vi "_RT_CtrlLoop_DigitalAnalogueOutput.vi"(6 "ExpVar.lvclass":refnum<class "ExpVar.lvclass">, 8 "error in (no error)":errorcluster, 9 "safty":refnum<data-value>) -> ()   [LabVIEW 2018]
uses:
  PublicSubVI/NewExpVar/ExpVar.lvclass
  PublicSubVI/Ctl/_ctl_RT_FPGA_Function.ctl
  PublicSubVI/Ctl/_ctl_RT_extDO.ctl
  PublicSubVI/Ctl/_ctl_RT_ExtAO.ctl
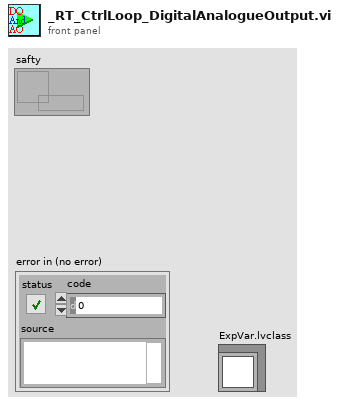
[diagram p1: front panel]
types:
  T1 = enum16{"None", "D999", "ExtAO", "ExtDO", "ExtDI_Label", "Signal_Remarks", "Script"}
  T2 = typedef "_ctl_RT_FPGA_Function.ctl" = enum16{"Initialisation", "Execution", "Digital In"}
  T3 = enum16{"via string label", "Laser", "Pressure", "TMP", "Script", "Signal Remarks", "ExtAO", "ExtDO", "ExtDI", "D999"}
  T4 = typedef "_ctl_RT_extDO.ctl" = cluster{"Label":string, "Boolean":bool}[]
  T5 = typedef "_ctl_RT_ExtAO.ctl" = cluster{"Label":string, "y":dbl}[]
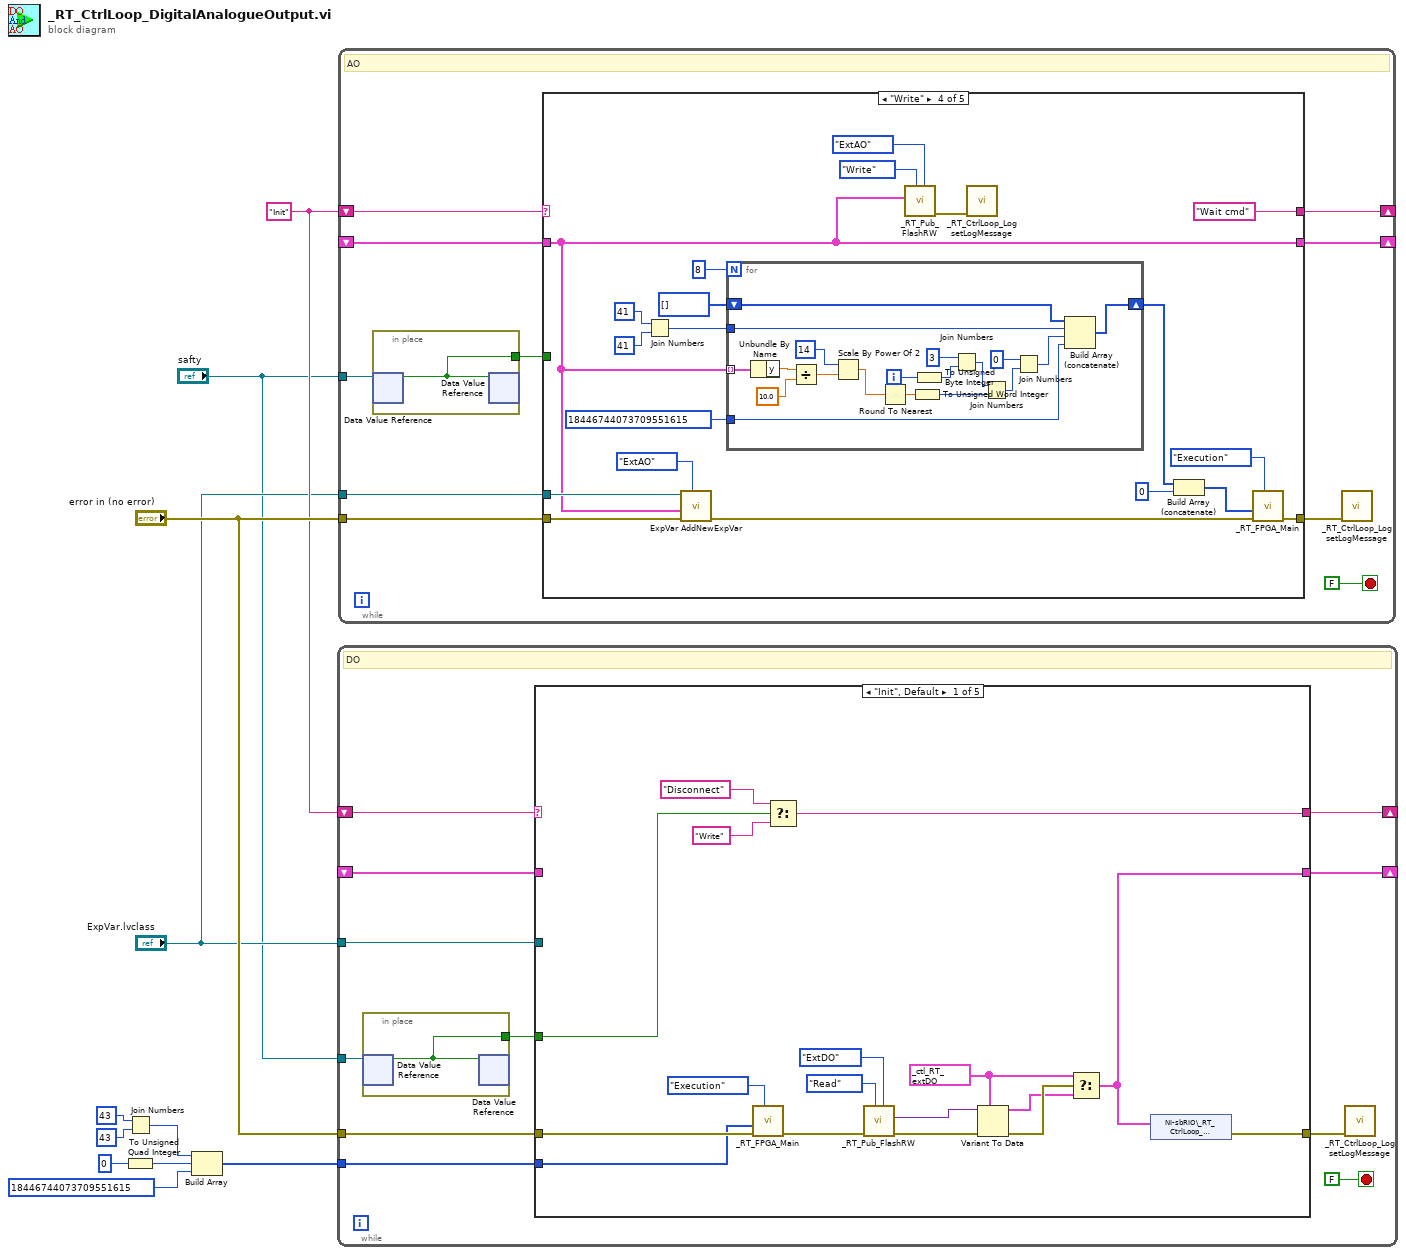
[diagram p0: block diagram]
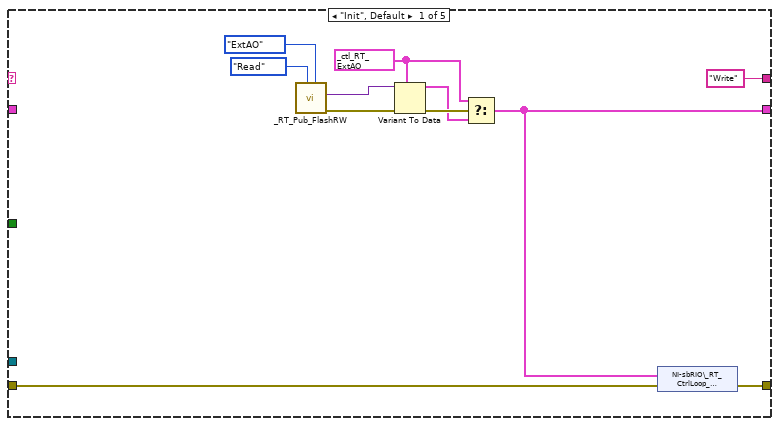
[diagram p2: hidden frame]
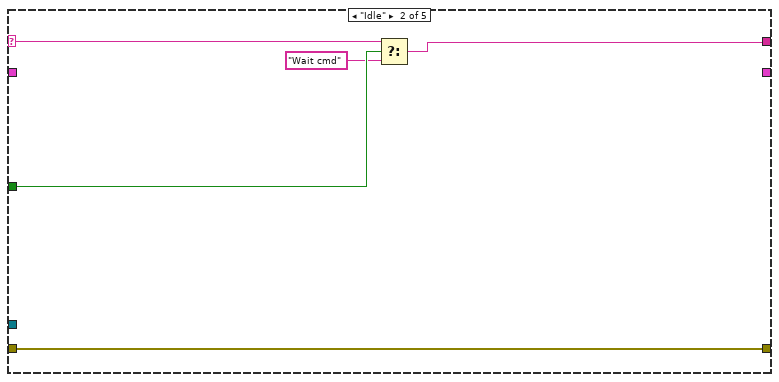
[diagram p3: hidden frame]
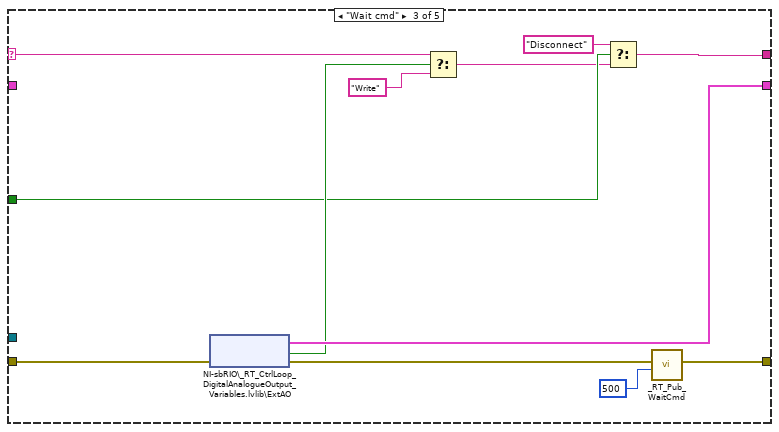
[diagram p4: hidden frame]
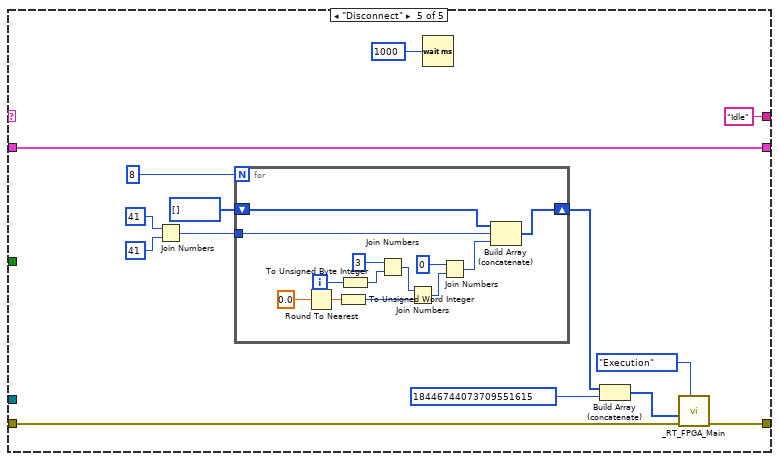
[diagram p5: hidden frame]
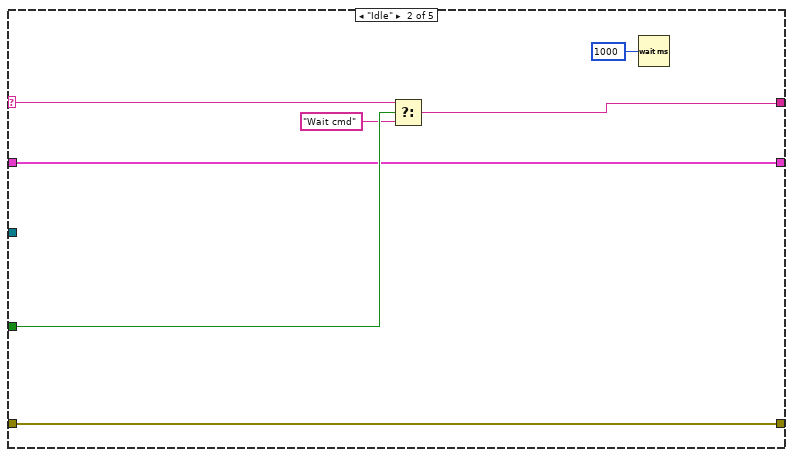
[diagram p6: hidden frame]
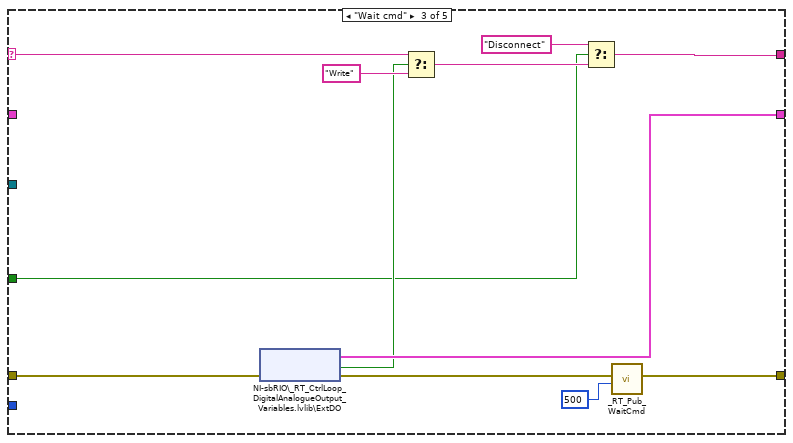
[diagram p7: hidden frame]
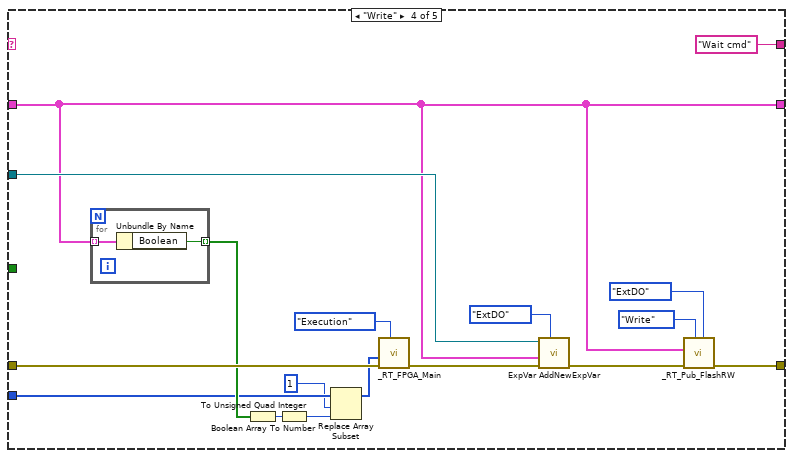
[diagram p8: hidden frame]
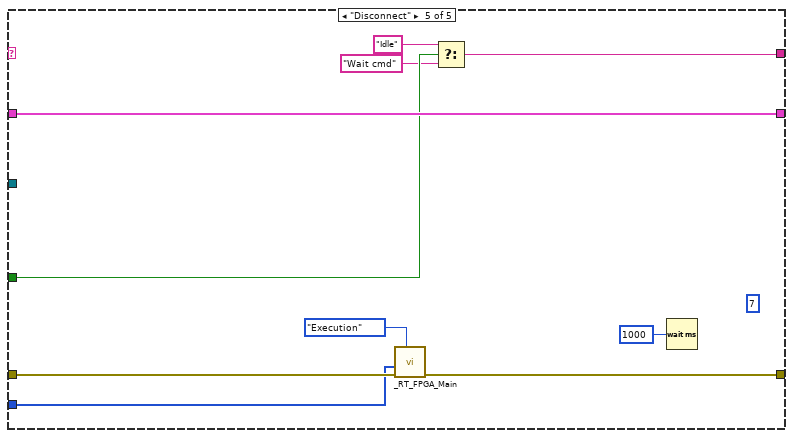
[diagram p9: hidden frame]
diagram:
  w3 = "Init"
  n1 = To Unsigned Quad Integer(1:u64 0 ("number")) -> (0:w7:u64)
  n2 = Join Numbers(hi=u32 43, lo=u32 43) -> ((hi.lo)=w10:u64)
  n3 = Build Array(w10, w7, u64 18446744073709551615 ("element")) -> (w4:u64[])
  n4 = while {
    shift-right: [w17] -> _
    shift-left: w3 -> [w19]
    shift-right: [w22] -> _
    shift-left: _ -> [w21]
    tunnel: "error in (no error)" -> [w20]
    tunnel: w4 -> [w16]
    tunnel: "ExpVar.lvclass" -> [w15]
    tunnel: "safty" -> [w13]
    stop <- FALSE stop-if-true
    # "DO"
    n5 = in-place {
      in-place-border: [w23] -> w12
      n6 = in-place-dvr #1(w13) -> (w23:bool)  [unwired: 1 out]
      n7 = in-place-dvr #1(w23) -> ()  [unwired: 2 out]
    }
    n8 = case shown="\"Init\", Default" w19 {
      selector: w19 -> [_ w41 w51 _ _]
      tunnel: [w36 w46 w48 "Wait cmd" w83] -> w17
      tunnel: [w25 w45 w55 w63 w86] -> w22
      tunnel: w21 -> [_ w45 _ w63 w86]
      tunnel: w20 -> [w35 w44 w59 w74 w87]
      tunnel: [w39 w44 w58 w61 w84] -> w14
      tunnel: w16 -> [w34 _ _ w71 w85]
      tunnel: w15 -> [_ _ _ w67 _]
      tunnel: w12 -> [w24 w47 w49 _ w80]
      frame "Init", Default {
        w26 = T4 [{"Label"="DO0", "Boolean"=FALSE}, {"Label"="DO1", "Boolean"=FALSE}, {"Label"="DO2", "Boolean"=FALSE}, {"Label"="DO3", "Boolean"=FALSE}, {"Label"="DO4", "Boolean"=FALSE}, {"Label"="DO5", "Boolean"=FALSE}, {"Label"="DO6", "Boolean"=FALSE}, {"Label"="DO7", "Boolean"=FALSE}] ("DOs")
        n9 = call "_RT_FPGA_Main.vi"("Function"=_ctl_RT_FPGA_Function."Execution", "Error in"=w35, "U64EventCodes"=w34) -> ("Error out"=w32:errorcluster)  [unwired: 6 in, 2 out]
        n10 = Select(t="Disconnect", s=w24, f="Write") -> (s? t:f=w36:string)
        n11 = call "_RT_Pub_FlashRW.vi"("FileEnum"=T1."ExtDO", "State"=enum16{"Read", "Write"}."Read", "error in (no error)"=w32) -> ("error out"=w30:errorcluster, "Value"=w31:variant)  [unwired: 6 in, 1 out]
        n12 = Variant To Data(error in=w30, type=w26, Variant=w31) -> (data=w27:T4, error out=w28:errorcluster)
        n13 = Select(t=w26, s=w28, f=w27) -> (s? t:f=w25:T4)
        n14 = shared-variable "NI-sbRIO\\_RT_CtrlLoop_DigitalAnalogueOutput_Variables.lvlib\\ExtDO"(w25) -> (error out=w39:errorcluster)  [unwired: 1 in]
      }
      frame "Idle" {
        n15 = Select(t=w41, s=w47, f="Wait cmd") -> (s? t:f=w46:string)
        n16 = Wait (ms)(milliseconds to wait=u32 1000) -> ()  [unwired: 1 out]
      }
      frame "Wait cmd" {
        n17 = shared-variable "NI-sbRIO\\_RT_CtrlLoop_DigitalAnalogueOutput_Variables.lvlib\\ExtDO"(error in=w59) -> (w55:T4, error out=w57:errorcluster, w50:bool)  [unwired: 1 in]
        n18 = Select(t=w51, s=w50, f="Write") -> (s? t:f=w52:string)
        n19 = Select(t="Disconnect", s=w49, f=w52) -> (s? t:f=w48:string)
        n20 = call "_RT_Pub_WaitCmd.vi"("milliseconds to wait"=u32 500, "error in (no error)"=w57) -> ("error out"=w58:errorcluster)  [unwired: 9 in]
      }
      frame "Write" {
        n21 = for {
          tunnel: w63 -> [w78] mode=indexing
          tunnel: [w77] -> w72 mode=indexing
          n22 = Unbundle By Name(w78) -> ("Boolean"=w77:bool)
        }
        n23 = Boolean Array To Number(Boolean array=w72) -> (number=w73:u32)
        n24 = To Unsigned Quad Integer(1:w73) -> (0:w69:u64)
        n25 = Replace Array Subset(array=w71, new element=w69, index=1) -> (w68:u64[])
        n26 = call "_RT_FPGA_Main.vi"("Function"=_ctl_RT_FPGA_Function."Execution", "Error in"=w74, "U64EventCodes"=w68) -> ("Error out"=w66:errorcluster)  [unwired: 6 in, 2 out]
        n27 = call-dynamic "ExpVar AddNewExpVar.vi"("VarType"=T3."ExtDO", "error in (no error)"=w66, "Var"=w63, "ExpVar in"=w67) -> ("error out"=w62:errorcluster)  [unwired: 6 in, 1 out]
        n28 = call "_RT_Pub_FlashRW.vi"("FileEnum"=T1."ExtDO", "State"=enum16{"Read", "Write"}."Write", "error in (no error)"=w62, "DataIn"=w63) -> ("error out"=w61:errorcluster)  [unwired: 5 in, 2 out]
      }
      frame "Disconnect" {
        (unwired) u16 7 ("N1")
        n29 = call "_RT_FPGA_Main.vi"("Function"=_ctl_RT_FPGA_Function."Execution", "Error in"=w87, "U64EventCodes"=w85) -> ("Error out"=w84:errorcluster)  [unwired: 6 in, 2 out]
        n30 = Select(t="Idle", s=w80, f="Wait cmd") -> (s? t:f=w83:string)
        n31 = Wait (ms)(milliseconds to wait=u32 1000) -> ()  [unwired: 1 out]
      }
    }
    n32 = call "_RT_CtrlLoop_Log setLogMessage.vi"("error in"=w14) -> ()  [unwired: 9 in, 2 out]
  }
  n33 = while {
    shift-right: [w93] -> _
    shift-left: w3 -> [w98]
    shift-right: [w97] -> _
    shift-left: _ -> [w96]
    tunnel: "error in (no error)" -> [w95]
    tunnel: "ExpVar.lvclass" -> [w92]
    tunnel: "safty" -> [w90]
    stop <- FALSE stop-if-true
    # "AO"
    n34 = in-place {
      in-place-border: [w99] -> w89
      n35 = in-place-dvr #2(w90) -> (w99:bool)  [unwired: 1 out]
      n36 = in-place-dvr #2(w99) -> ()  [unwired: 2 out]
    }
    n37 = case shown="\"Write\"" w98 {
      selector: w98 -> [_ w114 w120 _ _]
      tunnel: ["Write" w112 w116 "Wait cmd" "Idle"] -> w93
      tunnel: [w101 _ w126 w132 w170] -> w97
      tunnel: w96 -> [_ _ _ w132 w170]
      tunnel: w95 -> [w109 w111 w127 w136 w169]
      tunnel: [w110 w111 w125 w138 w171] -> w91
      tunnel: w92 -> [_ _ _ w135 _]
      tunnel: w89 -> [_ w115 w119 _ _]
      frame "Init", Default {
        w103 = T5 [{"Label"="AO0", "y"=0.0}, {"Label"="AO1", "y"=0.0}, {"Label"="AO2", "y"=0.0}, {"Label"="AO3", "y"=0.0}, {"Label"="AO4", "y"=0.0}, {"Label"="AO5", "y"=0.0}, {"Label"="AO6", "y"=0.0}, {"Label"="AO7", "y"=0.0}] ("ExtAO")
        n38 = call "_RT_Pub_FlashRW.vi"("FileEnum"=T1."ExtAO", "State"=enum16{"Read", "Write"}."Read") -> ("error out"=w106:errorcluster, "Value"=w107:variant)  [unwired: 7 in, 1 out]
        n39 = Variant To Data(error in=w106, type=w103, Variant=w107) -> (data=w102:T5, error out=w104:errorcluster)
        n40 = Select(t=w103, s=w104, f=w102) -> (s? t:f=w101:T5)
        n41 = shared-variable "NI-sbRIO\\_RT_CtrlLoop_DigitalAnalogueOutput_Variables.lvlib\\ExtAO"(w101, error in=w109) -> (error out=w110:errorcluster)
      }
      frame "Idle" {
        n42 = Select(t=w114, s=w115, f="Wait cmd") -> (s? t:f=w112:string)
      }
      frame "Wait cmd" {
        n43 = shared-variable "NI-sbRIO\\_RT_CtrlLoop_DigitalAnalogueOutput_Variables.lvlib\\ExtAO"(error in=w127) -> (w126:T5, error out=w121:errorcluster, w123:bool)  [unwired: 1 in]
        n44 = Select(t=w120, s=w123, f="Write") -> (s? t:f=w117:string)
        n45 = Select(t="Disconnect", s=w119, f=w117) -> (s? t:f=w116:string)
        n46 = call "_RT_Pub_WaitCmd.vi"("milliseconds to wait"=u32 500, "error in (no error)"=w121) -> ("error out"=w125:errorcluster)  [unwired: 9 in]
      }
      frame "Write" {
        n47 = Join Numbers(hi=u32 41, lo=u32 41) -> ((hi.lo)=w142:u64)
        n48 = call-dynamic "ExpVar AddNewExpVar.vi"("VarType"=T3."ExtAO", "error in (no error)"=w136, "Var"=w132, "ExpVar in"=w135) -> ("error out"=w137:errorcluster)  [unwired: 6 in, 1 out]
        n49 = for {
          N: 8 -> [_]
          tunnel: w142 -> [w166]
          tunnel: w132 -> [w156] mode=indexing
          shift-right: [w161] -> w140
          shift-left: u64[] [] -> [w160]
          tunnel: u64 18446744073709551615 ("element") -> [w148]
          i -> [w165]
          n50 = Unbundle By Name(w156) -> ("y"=w155:dbl)
          n51 = Divide(x=w155, y=10.0) -> (x/y=w153:dbl)
          n52 = Scale By Power Of 2(n=i16 14, x=w153) -> (x*2^n=w149:dbl)
          n53 = Round To Nearest(number=w149) -> (nearest integer value=w151:dbl)
          n54 = To Unsigned Word Integer(number=w151) -> (unsigned 16bit integer=w150:u16)
          n55 = To Unsigned Byte Integer(number=w165) -> (unsigned 8bit integer=w158:u8)
          n56 = Join Numbers(hi=u8 3, lo=w158) -> ((hi.lo)=w159:u16)
          n57 = Join Numbers(hi=w159, lo=w150) -> ((hi.lo)=w164:u32)
          n58 = Join Numbers(hi=u32 0, lo=w164) -> ((hi.lo)=w162:u64)
          n59 = Build Array (concatenate)(w160, w166, w162, w148) -> (w161:u64[])
        }
        n60 = call "_RT_Pub_FlashRW.vi"("FileEnum"=T1."ExtAO", "State"=enum16{"Read", "Write"}."Write", "DataIn"=w132) -> ("error out"=w128:errorcluster)  [unwired: 6 in, 2 out]
        n61 = call "_RT_CtrlLoop_Log setLogMessage.vi"("error in"=w128) -> ()  [unwired: 9 in, 2 out]
        n62 = Build Array (concatenate)(w140, u64 0) -> (w139:u64[])
        n63 = call "_RT_FPGA_Main.vi"("Function"=_ctl_RT_FPGA_Function."Execution", "Error in"=w137, "U64EventCodes"=w139) -> ("Error out"=w138:errorcluster)  [unwired: 6 in, 2 out]
      }
      frame "Disconnect" {
        n64 = Join Numbers(hi=u32 41, lo=u32 41) -> ((hi.lo)=w176:u64)
        n65 = for {
          N: 8 -> [_]
          tunnel: w176 -> [w193]
          shift-right: [w188] -> w174
          shift-left: u64[] [] -> [w187]
          i -> [w192]
          n66 = Round To Nearest(number=0.0) -> (nearest integer value=w183:dbl)
          n67 = To Unsigned Word Integer(number=w183) -> (unsigned 16bit integer=w182:u16)
          n68 = To Unsigned Byte Integer(number=w192) -> (unsigned 8bit integer=w185:u8)
          n69 = Join Numbers(hi=u8 3, lo=w185) -> ((hi.lo)=w186:u16)
          n70 = Join Numbers(hi=w186, lo=w182) -> ((hi.lo)=w191:u32)
          n71 = Join Numbers(hi=u32 0, lo=w191) -> ((hi.lo)=w189:u64)
          n72 = Build Array (concatenate)(w187, w193, w189) -> (w188:u64[])
        }
        n73 = Wait (ms)(milliseconds to wait=u32 1000) -> ()  [unwired: 1 out]
        n74 = Build Array (concatenate)(w174, u64 18446744073709551615 ("element")) -> (w173:u64[])
        n75 = call "_RT_FPGA_Main.vi"("Function"=_ctl_RT_FPGA_Function."Execution", "Error in"=w169, "U64EventCodes"=w173) -> ("Error out"=w171:errorcluster)  [unwired: 6 in, 2 out]
      }
    }
    n76 = call "_RT_CtrlLoop_Log setLogMessage.vi"("error in"=w91) -> ()  [unwired: 9 in, 2 out]
  }
